vi "Configure VSA.vi"(0 "instrument handle in":refnum<k21>, 2 "measurement interval (s)":dbl=0.001 format="%.2p", 3 "reference level":dbl format="%.2f", 4 "carrier frequency":dbl, 5 "error in":errorcluster, 6 "Selector String":string, 9 "RBW Filter Type":i32(ring)=2 items=["None"=5, "Gaussian"=1, "Flat"=2, "RRC"=6], 10 "RBW (Hz)":dbl=5000000.0 format="%.3p", 11 "RRC Alpha":dbl=0.1 format="%.2f") -> (14 "instrument handle out":refnum<k21>, 19 "error out":errorcluster)   [LabVIEW 2023]
uses:
  <vilib>/RFmx/SpecAn/mx/RFmxSpecAn.llb/RFmxSpecAn Select Measurement (Single).vi
  <resource>/objmgr/RFmxSpecAn.rc
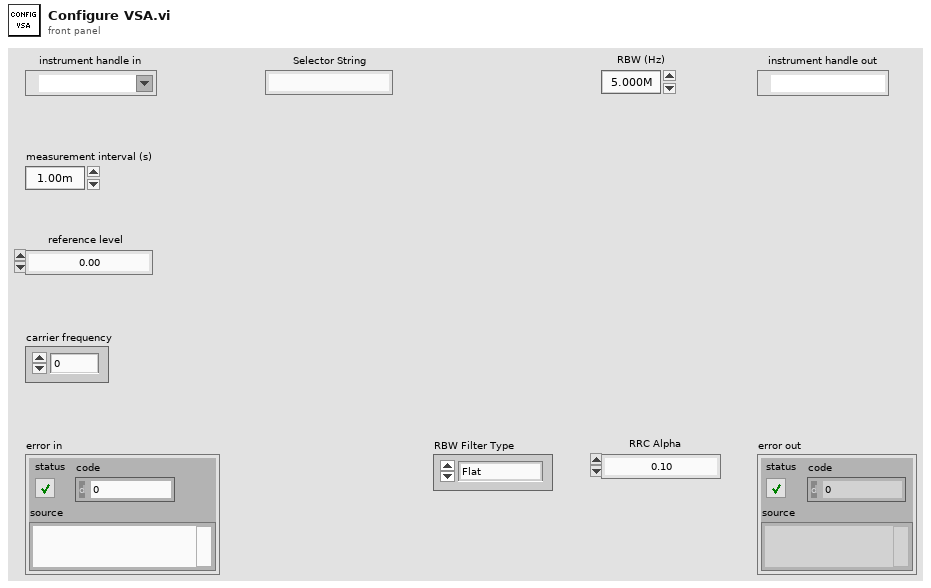
[diagram p1: front panel]
types:
  T1 = enum16{"ACP", "CCDF", "CHP", "FCnt", "Harmonics", "OBW", "SEM", "Spectrum", "Spur", "TXP", "AMPM", "DPD", "IQ", "IM", "NF", "PhaseNoise"}
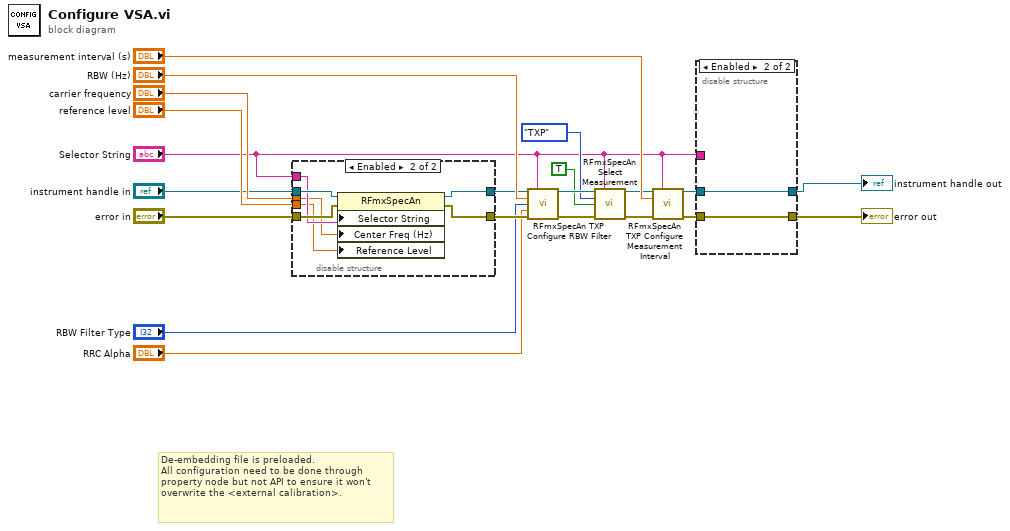
[diagram p0: block diagram]
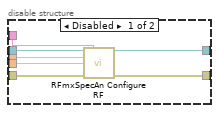
[diagram p2: hidden frame]
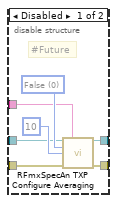
[diagram p3: hidden frame]
diagram:
  # "De-embedding file is preloaded.\nAll configuration need to be done through property node but not API to ensure it won't overwrite the <external calibration>."
  n1 = disable-structure shown="Enabled" {
    disable-tunnel: "error in" -> [w28 w32]
    disable-tunnel: [w27 w33] -> w20
    disable-tunnel: "carrier frequency" -> [w26 w30]
    disable-tunnel: "reference level" -> [w25 w29]
    disable-tunnel: "instrument handle in" -> [w24 w35]
    disable-tunnel: [w23 w34] -> w10
    disable-tunnel: "Selector String" -> [w22 w31]
    frame Disabled {
      n2 = call <vilib>:"RFmxSpecAn Configure RF.vi"("Instrument Handle In"=w24, "Selector String"=w22, "Center Frequency (Hz)"=w26, "Reference Level"=w25, "error in (no error)"=w28) -> ("Instrument Handle Out"=w23:refnum<k21>, "error out"=w27:errorcluster)  [unwired: 9 in]
    }
    frame Enabled {
      n3 = property class="RFmxSpecAn"(reference=w35, error in=w32, "Selector String"=w31, "Center Freq (Hz)"=w30, "Reference Level"=w29) -> (reference out=w34:refnum<k21>, error out=w33:errorcluster)
    }
  }
  n4 = call <vilib>:"RFmxSpecAn TXP Configure RBW Filter.vi"("Instrument Handle In"=w10, "Selector String"="Selector String", "RBW (Hz)"="RBW (Hz)", "RBW Filter Type"="RBW Filter Type", "RRC Alpha"="RRC Alpha", "error in (no error)"=w20) -> ("Instrument Handle Out"=w8:refnum<k21>, "error out"=w18:errorcluster)  [unwired: 8 in]
  n5 = call-poly <vilib>:"RFmxSpecAn Select Measurement.vi"("Instrument Handle In"=w8, "Selector String"="Selector String", "Measurement"=T1."TXP", "Enable All Traces"=TRUE, "error in (no error)"=w18) -> ("Instrument Handle Out"=w7:refnum<k21>, "error out"=w17:errorcluster)  [unwired: 9 in]
  n6 = call <vilib>:"RFmxSpecAn TXP Configure Measurement Interval.vi"("Instrument Handle In"=w7, "Selector String"="Selector String", "Measurement Interval (s)"="measurement interval (s)", "error in (no error)"=w17) -> ("Instrument Handle Out"=w9:refnum<k21>, "error out"=w19:errorcluster)  [unwired: 10 in]
  n7 = disable-structure shown="Enabled" {
    disable-tunnel: w19 -> [w42 w43]
    disable-tunnel: [w41 w43] -> w16
    disable-tunnel: w9 -> [w38 w44]
    disable-tunnel: [w37 w44] -> w3
    disable-tunnel: "Selector String" -> [w36 _]
    frame Disabled {
      w40 = 0 items=["False", "True"] ("Averaging Enabled")
      # "#Future"
      n8 = call <vilib>:"RFmxSpecAn TXP Configure Averaging.vi"("Instrument Handle In"=w38, "Selector String"=w36, "Averaging Enabled"=w40, "Averaging Count"=10, "error in (no error)"=w42) -> ("Instrument Handle Out"=w37:refnum<k21>, "error out"=w41:errorcluster)  [unwired: 9 in]
    }
    frame Enabled {
    }
  }
  "error out" <- w16
  "instrument handle out" <- w3
